vi "Main.vi"() -> ()   [LabVIEW 2024]
panel:
  in  "Mode":string
  in  "Position (degrees)":dbl
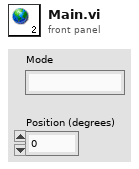
[diagram p1: front panel]
diagram:
